vi "8switchtermo.vi"() -> ()   [LabVIEW 2017]
panel:
  out "Meter":dbl(knob) scale=0.0..255.0
  out "Numeric 2":dbl format="%#_17g"
  out "Thermometer":dbl(slide) scale=0.0..255.0
  in  "stop":bool
  out "Array 2":dbl[](array[numeric])
  in  "Array":bool[](array[boolean])
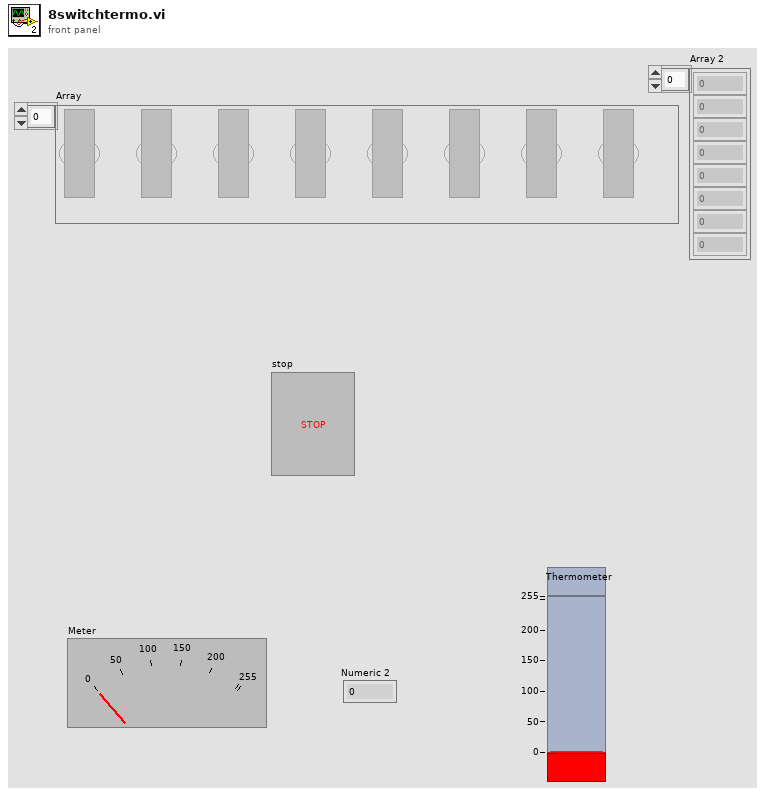
[diagram p1: front panel]
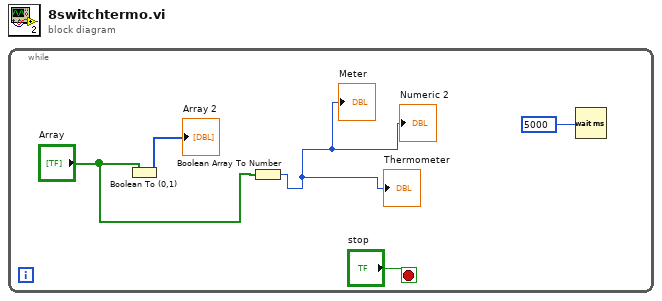
[diagram p0: block diagram]
diagram:
  n1 = while {
    stop <- "stop" stop-if-true
    n2 = Boolean To (0,1)(Boolean="Array") -> (0, 1=→"Array 2":i16[])
    n3 = Boolean Array To Number(Boolean array="Array") -> (number=→"Thermometer" →"Numeric 2" →"Meter":u32)
    n4 = Wait (ms)(milliseconds to wait=5000) -> ()  [unwired: 1 out]
  }
